vi "Write Position.vi"(3 "(FPSZ)":refnum<class "FPSZ.lvclass">, 4 "Position":T1) -> (5 "(FPSZ) Out":refnum<class "FPSZ.lvclass">)   [LabVIEW 2023, in "FPSZ.lvclass"]
uses:
  FPSZ.lvclass
  <vilib>/Utility/miscctls.llb/LVPositionTypeDef.ctl
  FPSZ.lvclass/FPSZ.ctl
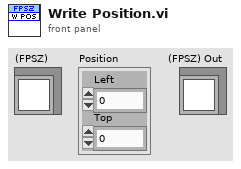
[diagram p1: front panel]
types:
  T1 = typedef "LVPositionTypeDef.ctl" = cluster{"Left":i32, "Top":i32}
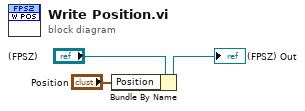
[diagram p0: block diagram]
diagram:
  n1 = Bundle By Name(cluster="(FPSZ)", "Position"="Position") -> (→"(FPSZ) Out":refnum<class "FPSZ.lvclass">)
